vi "Sensor de Pressao e Grafico.vi"() -> ()   [LabVIEW 2010]
uses:
  <vilib>/Analysis/3filter.llb/Filter Passband Type.ctl
  <vilib>/Analysis/3filter.llb/Butterworth Filter (DBL).vi
  <vilib>/LabVIEW Interface for Arduino/LabVIEW Interface for Arduino.lvlib
  <vilib>/Analysis/NI_AAL_SigProc.lvlib
  <vilib>/Analysis/NI_AALBase.lvlib
panel:
  out "Tempo para Amostragem":i32
  out "BPM":i32
  out "Gráfico de Frequência de Pulso":dbl[](graph)
  in  "Entrada Pino Analógico":u8
  in  "Frequencia da Amostragem (HZ)":u16
  in  "Amostras a ler":u32
  in  "stop":bool
  # "4000"
  # "120000"
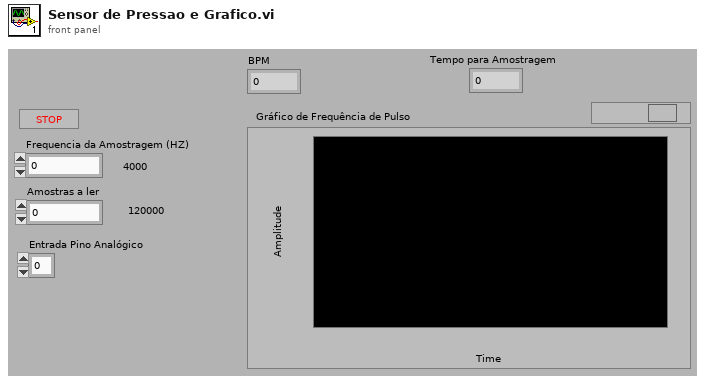
[diagram p1: front panel]
types:
  T1 = typedef "LabVIEW Interface for Arduino.lvlib/Arduino Resource.ctl" = cluster{"VISA resource":refnum<visa-resource-name>, "Board Type":T2, "Connection Type":enum8{"USB / Serial"}, "Bytes Per Packet (15)":u8}
  T2 = typedef "LabVIEW Interface for Arduino.lvlib/Board Type.ctl" = enum16{"Uno", "Dimuelanove w/Atmega 328", "Mega 2560"}
  T3 = typedef "NI_AALBase.lvlib/Filter Passband Type.ctl" = enum32{"Lowpass", "Highpass", "Bandpass", "Bandstop"}
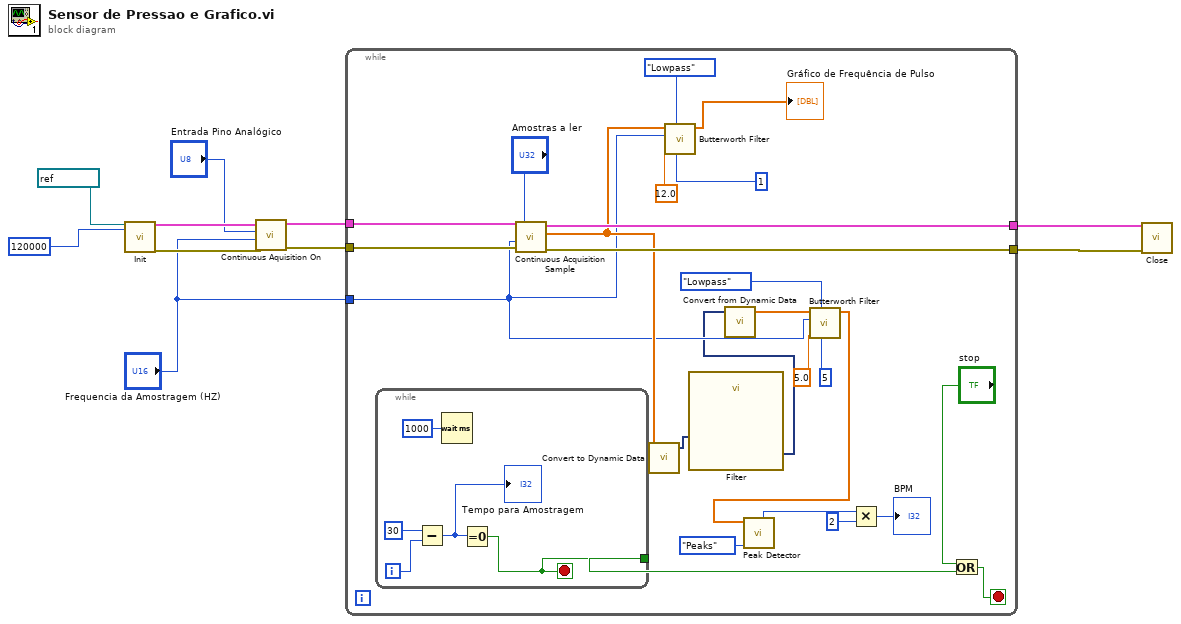
[diagram p0: block diagram]
diagram:
  n1 = call <vilib>:"Init.vi"("VISA resource"=refnum<visa-resource-name> "COM5", "Baud Rate (115200)"=u32 120000) -> ("Arduino Resource"=w10:T1, "error out"=w9:errorcluster)  [unwired: 16 in]
  n2 = call <vilib>:"Continuous Aquisition On.vi"("error in"=w9, "Acquition Speed"="Frequencia da Amostragem (HZ)", "Analog Input Pin"="Entrada Pino Analógico", "Arduino Resource"=w10) -> ("error out"=w7:errorcluster, "Arduino Resource"=w8:T1)  [unwired: 6 in]
  n3 = while {
    tunnel: w8 -> [w35]
    tunnel: w7 -> [w34]
    tunnel: [w32] -> w6
    tunnel: [w31] -> w5
    tunnel: "Frequencia da Amostragem (HZ)" -> [w23]
    stop <- w14 stop-if-true
    n4 = while {
      tunnel: [w37] -> w13
      i -> [w40]
      stop <- w37 stop-if-true
      n5 = Subtract(x=30, y=w40) -> (x-y=w39:i32)
      "Tempo para Amostragem" <- w39
      n6 = Wait (ms)(milliseconds to wait=u32 1000) -> ()  [unwired: 1 out]
      n7 = Equal To 0?(x=w39) -> (x = 0?=w37:bool)
    }
    n8 = call <vilib>:"Continuous Acquisition Sample.vi"("Arduino Resource"=w35, "Samples to Read"="Amostras a ler", "Sample Rate (HZ)"=w23, "error in (no error)"=w34) -> ("Arduino Resource"=w32:T1, "Data"=w26:dbl[], "error out"=w31:errorcluster)  [unwired: 4 in]
    n9 = call "Convert to Dynamic Data"("Array"=w26) -> ("Dynamic Data Type"=w12:dynamicdata)  [unwired: 3 in]
    n10 = call-poly <vilib>:"Butterworth Filter.vi"("order"=1, "filter type"=Filter_Passband_Type."Lowpass", "low cutoff freq: fl"=12.0, "sampling freq: fs"=w23, "X"=w26) -> ("Filtered X"=→"Gráfico de Frequência de Pulso":dbl[])  [unwired: 3 in, 1 out]
    n11 = call "Filter"("Signal"=w12) -> ("Filtered Signal"=w11:dynamicdata)  [unwired: 9 in, 1 out]
    n12 = call "Convert from Dynamic Data"("Dynamic Data Type"=w11) -> ("Array"=w25:dbl[])  [unwired: 3 in]
    n13 = call-poly <vilib>:"Butterworth Filter.vi"("order"=5, "filter type"=Filter_Passband_Type."Lowpass", "low cutoff freq: fl"=5.0, "sampling freq: fs"=w23, "X"=w25) -> ("Filtered X"=w19:dbl[])  [unwired: 3 in, 1 out]
    n14 = call <vilib>:"Peak Detector.vi"("peaks/valleys"=enum32{"Peaks", "Valleys"}."Peaks", "X"=w19) -> ("# found"=w18:i32)  [unwired: 5 in, 4 out]
    n15 = Multiply(x=w18, y=2) -> (x*y=→"BPM":i32)
    n16 = Or(x="stop", y=w13) -> (x .or. y?=w14:bool)
  }
  n17 = call <vilib>:"Close.vi"("Arduino Resource"=w6, "error in"=w5) -> ()  [unwired: 13 in, 1 out]
